vi "Master VI.vi"() -> ()   [LabVIEW 2020]
uses:
  <vilib>/Platform/browser.llb/Open URL in Default Browser (string).vi
  MainVIs.lvlib
  AnalysisSupport.lvlib
  <resource>/objmgr/daqmx.rc
panel:
  in  "Stenosis Testing":bool
  in  "Fix LVM Button":bool
  in  "Extract F0":bool
  in  "Extract Button":bool
  in  "Report Error or Request Change":bool
  in  "SPL":bool
  in  "Calibration":bool
  in  "Analysis":bool
  in  "Clipper":bool
  in  "Singing Helmet":bool
  in  "Redirect":bool
  in  "Complete":bool
  in  "Exit Button":bool
  in  "Incomplete":bool
  # "Select a Program"
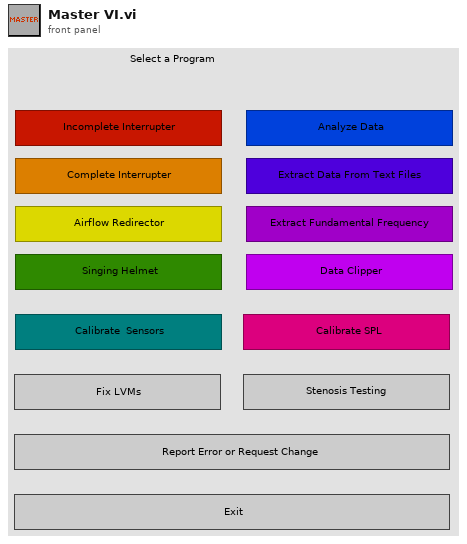
[diagram p1: front panel]
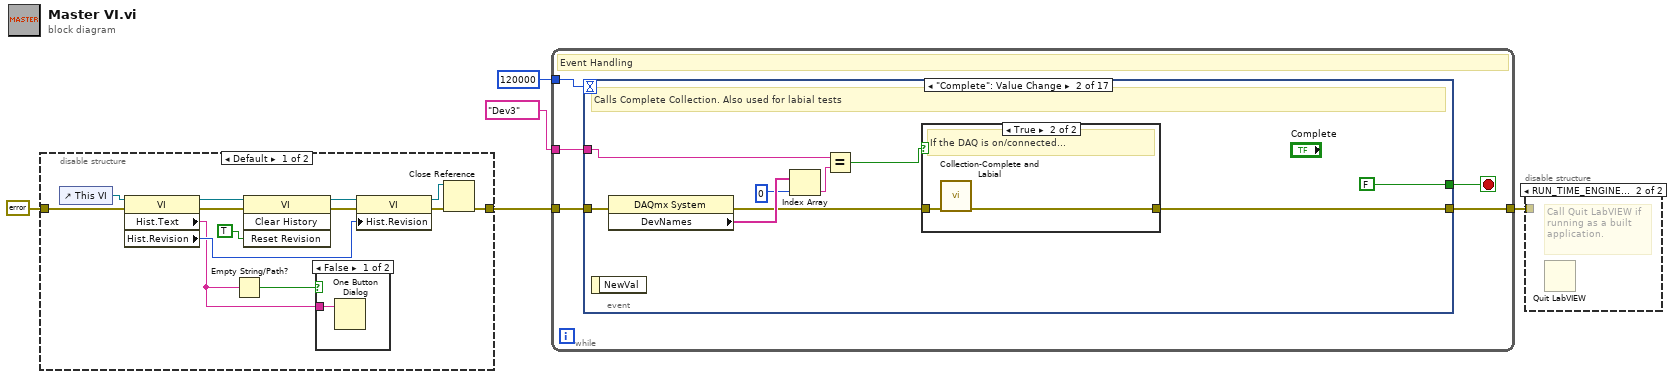
[diagram p0: block diagram]
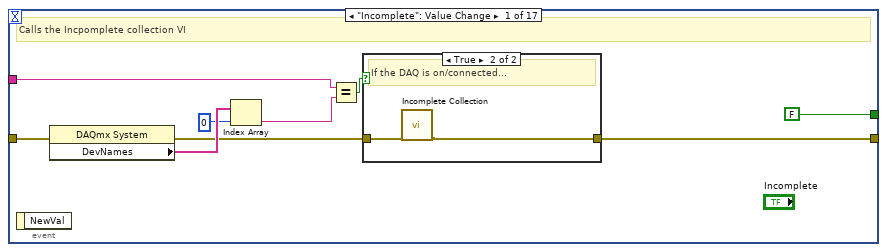
[diagram p5: hidden frame]
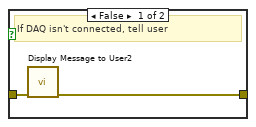
[diagram p6: hidden frame]
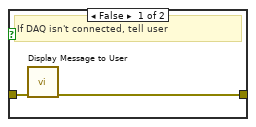
[diagram p7: hidden frame]
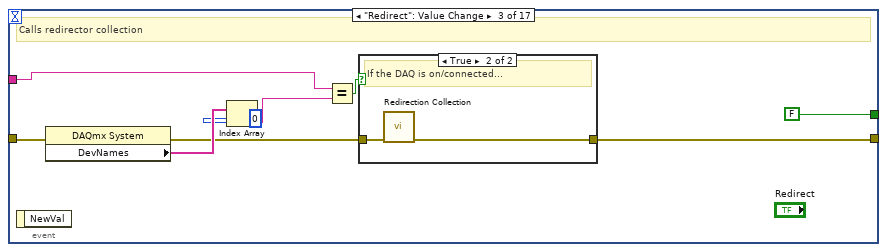
[diagram p8: hidden frame]
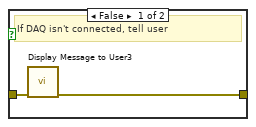
[diagram p9: hidden frame]
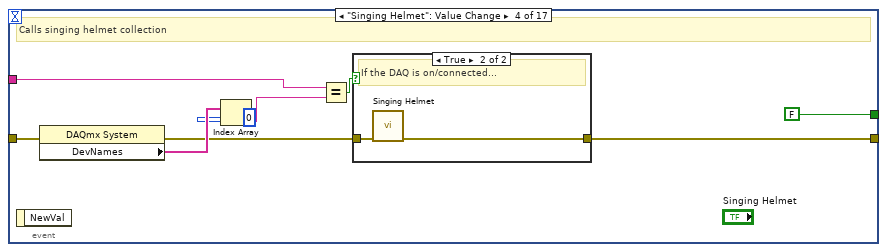
[diagram p10: hidden frame]
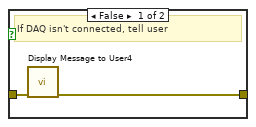
[diagram p11: hidden frame]
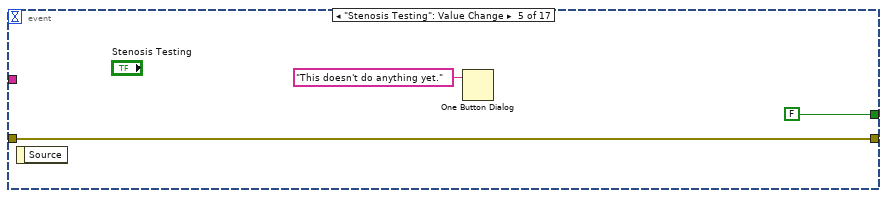
[diagram p12: hidden frame]
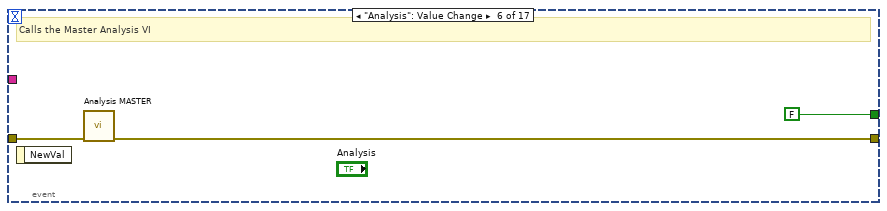
[diagram p13: hidden frame]
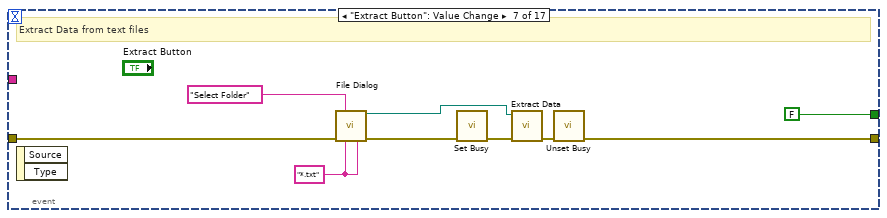
[diagram p14: hidden frame]
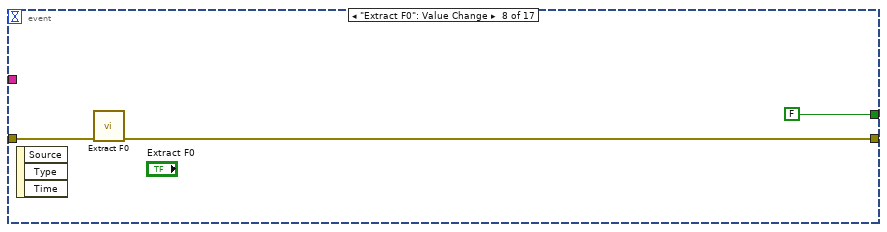
[diagram p15: hidden frame]
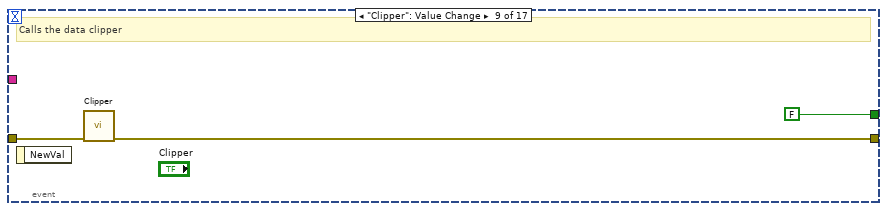
[diagram p16: hidden frame]
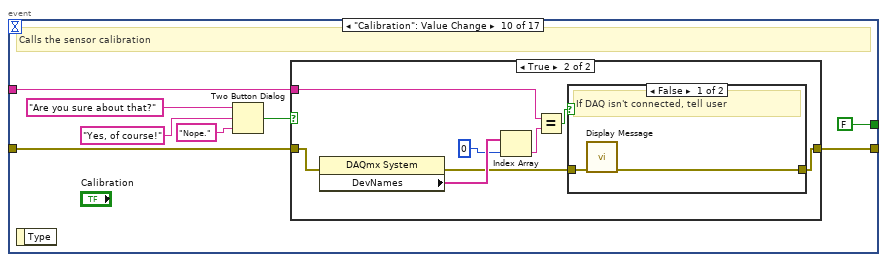
[diagram p17: hidden frame]
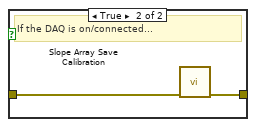
[diagram p19: hidden frame]
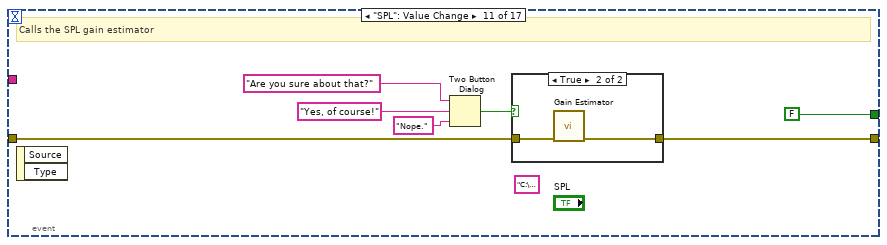
[diagram p20: hidden frame]
diagram:
  n1 = disable-structure "Conditional Disable Structure" shown="Default" {
    disable-tunnel: errorcluster {"status"=FALSE, "code"=0, "source"=""} ("error constant") -> [w7 w20]
    disable-tunnel: [w6 w20] -> w1
    frame condition #0 (active) {
      n2 = control-ref of="This VI"() -> (w11:refnum<vi>)
      n3 = property class="VI"(reference=w11, error in=w7) -> (reference out=w9:refnum<vi>, error out=w10:errorcluster, "Hist.Text"=w12:string, "Hist.Revision"=w18:u32)
      n4 = Empty String/Path?(string/path=w12) -> (empty?=w13:bool)
      n5 = invoke class="VI" method="Clear History"(reference=w9, error in=w10, "Reset Revision"=TRUE) -> (reference out=w14:refnum<vi>, error out=w15:errorcluster)  [unwired: 1 in, 2 out]
      n6 = case shown="False" w13 {
        tunnel: w12 -> [w19 _]
        frame False {
          n7 = One Button Dialog(message=w19) -> ()  [unwired: 1 in, 1 out]
        }
        frame True {
        }
      }
      n8 = property class="VI"(reference=w14, error in=w15, "Hist.Revision"=w18) -> (reference out=w16:refnum<vi>, error out=w17:errorcluster)
      n9 = Close Reference(reference=w16, error in (no error)=w17) -> (error out=w6:errorcluster)
    }
    frame condition #1 {
    }
  }
  n10 = while {
    tunnel: [w24] -> w5
    tunnel: w1 -> [w23]
    tunnel: 120000 -> [w22]
    tunnel: tag "Dev3" -> [w21]
    stop <- w25 stop-if-true
    # "Event Handling"
    n11 = event shown="[1] \"Complete\": Value Change" {
      selector: _ -> [_ _ _ _ _ _ _ _ _ _ _ _ _ _ _ _ _]
      dyn-events: _ -> [_ _ _ _ _ _ _ _ _ _ _ _ _ _ _ _ _]
      timeout: w22 -> [_ _ _ _ _ _ _ _ _ _ _ _ _ _ _ _ _]
      tunnel: [FALSE FALSE FALSE FALSE FALSE FALSE FALSE FALSE FALSE FALSE FALSE FALSE FALSE TRUE w146 TRUE TRUE] -> w25
      tunnel: [w27 w41 w53 w66 w80 w82 w85 w94 w97 w105 w125 w132 w137 w144 w148 w150 w153] -> w24
      tunnel: w23 -> [w28 w40 w54 w67 w80 w83 w89 w95 w98 w106 w126 w133 w136 w144 w149 w150 w153]
      tunnel: w21 -> [w26 w39 w52 w65 _ _ _ _ _ w99 _ _ _ _ _ _ _]
      event "Incomplete": Value Change {
        # "Calls the Incpomplete collection VI"
        n12 = event-data() -> ()  [unwired: 1 in, 1 out]
        n13 = property class="DAQmx System"(error in=w28) -> (error out=w32:errorcluster, "DevNames"=w33:tag[])  [unwired: 1 in, 1 out]
        n14 = Index Array(array=w33, index=0) -> (element=w31:tag)
        n15 = Equal?(x=w26, y=w31) -> (x = y?=w30:bool)
        n16 = case shown="True" w30 {
          tunnel: w32 -> [w36 w38]
          tunnel: [w35 w37] -> w27
          frame False {
            # "If DAQ isn't connected, tell user"
            n17 = call "Display Message to User2"("error in (no error)"=w36) -> ("error out"=w35:errorcluster)  [unwired: 9 in, 1 out]
          }
          frame True {
            # "If the DAQ is on/connected..."
            n18 = call "Incomplete Collection.vi"("error in (no error)"=w38) -> ("error out"=w37:errorcluster)  [unwired: 10 in]
          }
        }
      }
      event "Complete": Value Change {
        # "Calls Complete Collection. Also used for labial tests"
        n19 = event-data() -> ()  [unwired: 1 in, 1 out]
        n20 = property class="DAQmx System"(error in=w40) -> (error out=w45:errorcluster, "DevNames"=w46:tag[])  [unwired: 1 in, 1 out]
        n21 = Index Array(array=w46, index=0) -> (element=w44:tag)
        n22 = Equal?(x=w39, y=w44) -> (x = y?=w43:bool)
        n23 = case shown="True" w43 {
          tunnel: w45 -> [w49 w51]
          tunnel: [w48 w50] -> w41
          frame False {
            # "If DAQ isn't connected, tell user"
            n24 = call "Display Message to User"("error in (no error)"=w49) -> ("error out"=w48:errorcluster)  [unwired: 9 in, 1 out]
          }
          frame True {
            # "If the DAQ is on/connected..."
            n25 = call "Collection-Complete and Labial.vi"("error in"=w51) -> ("error out"=w50:errorcluster)  [unwired: 10 in]
          }
        }
      }
      event "Redirect": Value Change {
        # "Calls redirector collection"
        n26 = event-data() -> ()  [unwired: 1 in, 1 out]
        n27 = property class="DAQmx System"(error in=w54) -> (error out=w58:errorcluster, "DevNames"=w59:tag[])  [unwired: 1 in, 1 out]
        n28 = Index Array(array=w59, index=0) -> (element=w57:tag)
        n29 = Equal?(x=w52, y=w57) -> (x = y?=w56:bool)
        n30 = case shown="True" w56 {
          tunnel: w58 -> [w62 w63]
          tunnel: [w61 w64] -> w53
          frame False {
            # "If DAQ isn't connected, tell user"
            n31 = call "Display Message to User3"("error in (no error)"=w62) -> ("error out"=w61:errorcluster)  [unwired: 9 in, 1 out]
          }
          frame True {
            # "If the DAQ is on/connected..."
            n32 = call "Redirection Collection.vi"("error in"=w63) -> ("error out"=w64:errorcluster)  [unwired: 10 in]
          }
        }
      }
      event "Singing Helmet": Value Change {
        # "Calls singing helmet collection"
        n33 = event-data() -> ()  [unwired: 1 in, 1 out]
        n34 = property class="DAQmx System"(error in=w67) -> (error out=w71:errorcluster, "DevNames"=w72:tag[])  [unwired: 1 in, 1 out]
        n35 = Index Array(array=w72, index=0) -> (element=w70:tag)
        n36 = Equal?(x=w65, y=w70) -> (x = y?=w69:bool)
        n37 = case shown="True" w69 {
          tunnel: w71 -> [w75 w77]
          tunnel: [w74 w76] -> w66
          frame False {
            # "If DAQ isn't connected, tell user"
            n38 = call "Display Message to User4"("error in (no error)"=w75) -> ("error out"=w74:errorcluster)  [unwired: 9 in, 1 out]
          }
          frame True {
            # "If the DAQ is on/connected..."
            n39 = call "Singing Helmet.vi"("error in (no error)"=w77) -> ("error out"=w76:errorcluster)  [unwired: 10 in]
          }
        }
      }
      event "Stenosis Testing": Value Change {
        n40 = event-data() -> ()  [unwired: 1 in, 1 out]
        n41 = One Button Dialog(message="This doesn't do anything yet.") -> ()  [unwired: 1 in, 1 out]
      }
      event "Analysis": Value Change {
        # "Calls the Master Analysis VI"
        n42 = event-data() -> ()  [unwired: 1 in, 1 out]
        n43 = call "Analysis MASTER.vi"("Error In"=w83) -> ("Error Out"=w82:errorcluster)  [unwired: 10 in]
      }
      event "Extract Button": Value Change {
        w91 = "*.txt" ("pattern label")
        # "Extract Data from text files"
        n44 = event-data() -> ()  [unwired: 1 in, 2 out]
        n45 = call "File Dialog"("prompt"="Select Folder", "error in"=w89, "pattern (all files)"=w91, "pattern label"=w91) -> ("selected path"=w90:path, "error out"=w88:errorcluster)  [unwired: 8 in, 2 out]
        n46 = call <vilib>:"Set Busy.vi"("error in (no error)"=w88) -> ("error out"=w87:errorcluster)  [unwired: 9 in, 1 out]
        n47 = call "Extract Data.vi"("Error In"=w87, "Folder Path"=w90) -> ("Error Out"=w86:errorcluster)  [unwired: 9 in]
        n48 = call <vilib>:"Unset Busy.vi"("error in (no error)"=w86) -> ("error out"=w85:errorcluster)  [unwired: 10 in]
      }
      event "Extract F0": Value Change {
        n49 = event-data() -> ()  [unwired: 1 in, 3 out]
        n50 = call "Extract F0.vi"("Error In"=w95) -> ("Error Out"=w94:errorcluster)  [unwired: 10 in]
      }
      event "Clipper": Value Change {
        # "Calls the data clipper"
        n51 = event-data() -> ()  [unwired: 1 in, 1 out]
        n52 = call "Clipper.vi"("error in (no error)"=w98) -> ("error out"=w97:errorcluster)  [unwired: 10 in]
      }
      event "Calibration": Value Change {
        # "Calls the sensor calibration"
        n53 = event-data() -> ()  [unwired: 1 in, 1 out]
        n54 = Two Button Dialog(message="Are you sure about that?", 1:"Nope." ("F button name (\"Cancel\")"), 2:"Yes, of course!" ("T button name (\"OK\")")) -> (T button?=w101:bool)
        n55 = case shown="True" w101 {
          tunnel: w106 -> [w107 w110]
          tunnel: [w107 w109] -> w105
          tunnel: w99 -> [_ w108]
          frame False {
          }
          frame True {
            n56 = property class="DAQmx System"(error in=w110) -> (error out=w114:errorcluster, "DevNames"=w115:tag[])  [unwired: 1 in, 1 out]
            n57 = Index Array(array=w115, index=0) -> (element=w113:tag)
            n58 = Equal?(x=w108, y=w113) -> (x = y?=w112:bool)
            n59 = case shown="False" w112 {
              tunnel: w114 -> [w117 w119]
              tunnel: [w116 w118] -> w109
              frame False {
                # "If DAQ isn't connected, tell user"
                n60 = call "Display Message"("error in (no error)"=w117) -> ("error out"=w116:errorcluster)  [unwired: 9 in, 1 out]
              }
              frame True {
                # "If the DAQ is on/connected..."
                n61 = call "Slope Array Save Calibration.vi"("Error In"=w119) -> ("Error Out"=w118:errorcluster)  [unwired: 11 in, 3 out]
              }
            }
          }
        }
      }
      event "SPL": Value Change {
        (unwired) "C:\\Program Files (x86)\\Audacity\\audacity.exe" ("command line")
        # "Calls the SPL gain estimator"
        n62 = event-data() -> ()  [unwired: 1 in, 2 out]
        n63 = Two Button Dialog(message="Are you sure about that?", 1:"Nope." ("F button name (\"Cancel\")"), 2:"Yes, of course!" ("T button name (\"OK\")")) -> (T button?=w121:bool)
        n64 = case shown="True" w121 {
          tunnel: w126 -> [w127 w129]
          tunnel: [w127 w128] -> w125
          frame False {
          }
          frame True {
            n65 = call "Gain Estimator.vi"("error in (no error)"=w129) -> ("Error Out"=w128:errorcluster)  [unwired: 8 in, 2 out]
          }
        }
      }
      event "Report Error or Request Change": Value Change {
        n66 = event-data() -> ()  [unwired: 1 in, 2 out]
        n67 = call-poly <vilib>:"Open URL in Default Browser.vi"("error in (no error)"=w133, "URL"="https://goo.gl/forms/o6MZTBsEczWoqA8r1") -> ("error out"=w132:errorcluster)  [unwired: 4 in, 1 out]
      }
      event "Fix LVM Button": Value Change {
        # "Runs the LVM Fixer"
        n68 = event-data() -> ()  [unwired: 1 in, 3 out]
        n69 = call "File Dialog - Fixer"("error in"=w136) -> ("selected path"=w139:path, "cancelled"=w135:bool, "error out"=w138:errorcluster)  [unwired: 11 in, 1 out]
        n70 = case shown="False" w135 {
          tunnel: w139 -> [w142 _]
          tunnel: w138 -> [w141 w143]
          tunnel: [w140 w143] -> w137
          frame False {
            n71 = call "Main.vi"("Error In"=w141, "Folder"=w142) -> ("Error Out"=w140:errorcluster)  [unwired: 9 in]
          }
          frame True {
          }
        }
      }
      event "Exit Button": Value Change {
        # "Exits the VI"
        n72 = event-data() -> ()  [unwired: 1 in, 1 out]
      }
      event Timeout {
        n73 = event-data() -> ()  [unwired: 1 in, 3 out]
        n74 = call "Timeout Check.vi"("Error In"=w149) -> ("Error Out"=w148:errorcluster, "Still there?"=w147:bool)  [unwired: 9 in]
        n75 = Not(x=w147) -> (.not. x?=w146:bool)
      }
      event Application Instance Close {
        # "The user has closed the app"
        n76 = event-data() -> ()  [unwired: 1 in, 1 out]
      }
      event Panel Close? {
        # "the panel has been closed"
        n77 = event-data() -> ()  [unwired: 1 in, 1 out]
        n78 = event-data() -> ()  [unwired: 2 in, 1 out]
      }
    }
  }
  n79 = disable-structure shown="RUN_TIME_ENGINE==True" {
    disable-tunnel: w5 -> [_ _]
    frame condition #0 (active) {
    }
    frame condition #1 {
      # "Call Quit LabVIEW if running as a built application."
      n80 = Quit LabVIEW() -> ()  [unwired: 1 in]
    }
  }
